vi "getGpsOptions.vi"(8 "error in (no error)":errorcluster, 11 "pHandle":u32) -> (0 "error out":errorcluster, 1 "return type":i32, 2 "pOptionsStr":string, 3 "pModelStr":string)   [LabVIEW 2011, in "sbgLabView.lvlib"]
uses:
  sbgLabView.lvlib
  sbgMatLab.dll
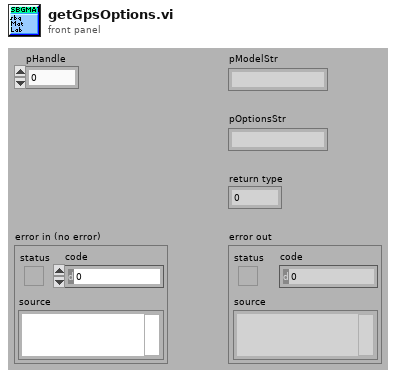
[diagram p1: front panel]
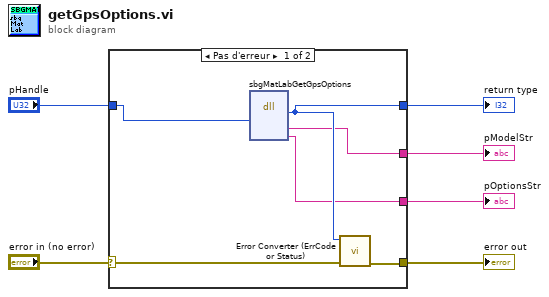
[diagram p0: block diagram]
diagram:
  n1 = case shown="Pas d'erreur" "error in (no error)" {
    selector: "error in (no error)" -> [w8 w13]
    tunnel: [w7 w13] -> w5
    tunnel: [w12 _] -> w4
    tunnel: "pHandle" -> [w11 _]
    tunnel: [w10 _] -> w2
    tunnel: [w9 _] -> w1
    frame No Error {
      n2 = dll-call lib="C:/SBG-Systems/remote/projects/software/projects/labviewExample/sbgLabView/sbgMatLab.*" fn="sbgMatLabGetGpsOptions"("pHandle"=w11) -> ("type de retour"=w12:i32, "modelStr"=w10:string, "optionsStr"=w9:string)  [unwired: 6 in, 2 out]
      n3 = call "Error Converter (ErrCode or Status).vi"("error in (no error)"=w8, "error code"=w12) -> ("error out"=w7:errorcluster)  [unwired: 9 in]
    }
    frame Error {
    }
  }
  "return type" <- w4
  "pModelStr" <- w2
  "pOptionsStr" <- w1
  "error out" <- w5
